vi "Autonomous Independent.vi"   [LabVIEW 2011]
doc: "This VI is called when autonomous begins, and will automatically be terminated when autonomous ends. You can carry out timed or sensor driven robot movement independently without needing to return to the caller."
uses:
  Robot Global Data.vi
types:
  T1 = typedef "WPI_JoystickDevRef.ctl" = cluster{"Device":T2}
  T2 = typedef "WPI_JoystickDeviceEnum.ctl" = enum16{"USB 1", "USB 2", "USB 3", "USB 4", "Kinect 1", "Kinect 2"}
  T3 = cluster{"axis 1 (x)":dbl, "axis 2 (y)":dbl, "axis 3 (throttle)":dbl, "axis 4":dbl, "axis 5":dbl, "axis 6":dbl}
  T4 = typedef "WPI_RobotDriveDevRef.ctl" = cluster{"DevStatus":errorcluster, "Motors[]":T5[], "Square Inputs":bool, "Max Output":dbl, "Isochronous":bool}
  T5 = typedef "WPI_MotorControlDeviceRef.ctl" = cluster{"DeviceStatus":errorcluster, "Type":enum16{"PWM", "CAN"}, "PWM":cluster{"Digital Module":T6, "PWM Channel":T7, "DeadBand":T8}, "CAN":cluster{"Device Number":u8, "Control Mode":T9, "Semaphore":T10, "Max Vout":dbl}, "Invert":bool, "TransformRef":T11, "InvTransformRef":T11}
  T6 = typedef "FPGA_TypedefDigitalModule.ctl" = enum16{"Digital Module 1", "Digital Module 2"}
  T7 = typedef "FPGA_DIOPWMChannel.ctl" = enum8{"PWM 1", "PWM 2", "PWM 3", "PWM 4", "PWM 5", "PWM 6", "PWM 7", "PWM 8", "PWM 9", "PWM 10", "Invalid"}
  T8 = typedef "WPI_PWMDeadband.ctl" = cluster{"Name":string, "maxPositivePwm":i32, "minPositivePwm":i32, "centerPwm":i32, "maxNegativePwm":i32, "minNegativePwm":i32, "angularRange":u16}
  T9 = typedef "WPI_CANJaguar_ControlMode.ctl" = enum8{"Percent VBus", "Current", "Speed", "Position", "Voltage"}
  T10 = typedef "Semaphore RefNum" = refnum<k1>
  T11 = typedef "WPI_PWMTransform_ConPane.ctl" = refnum<vi>
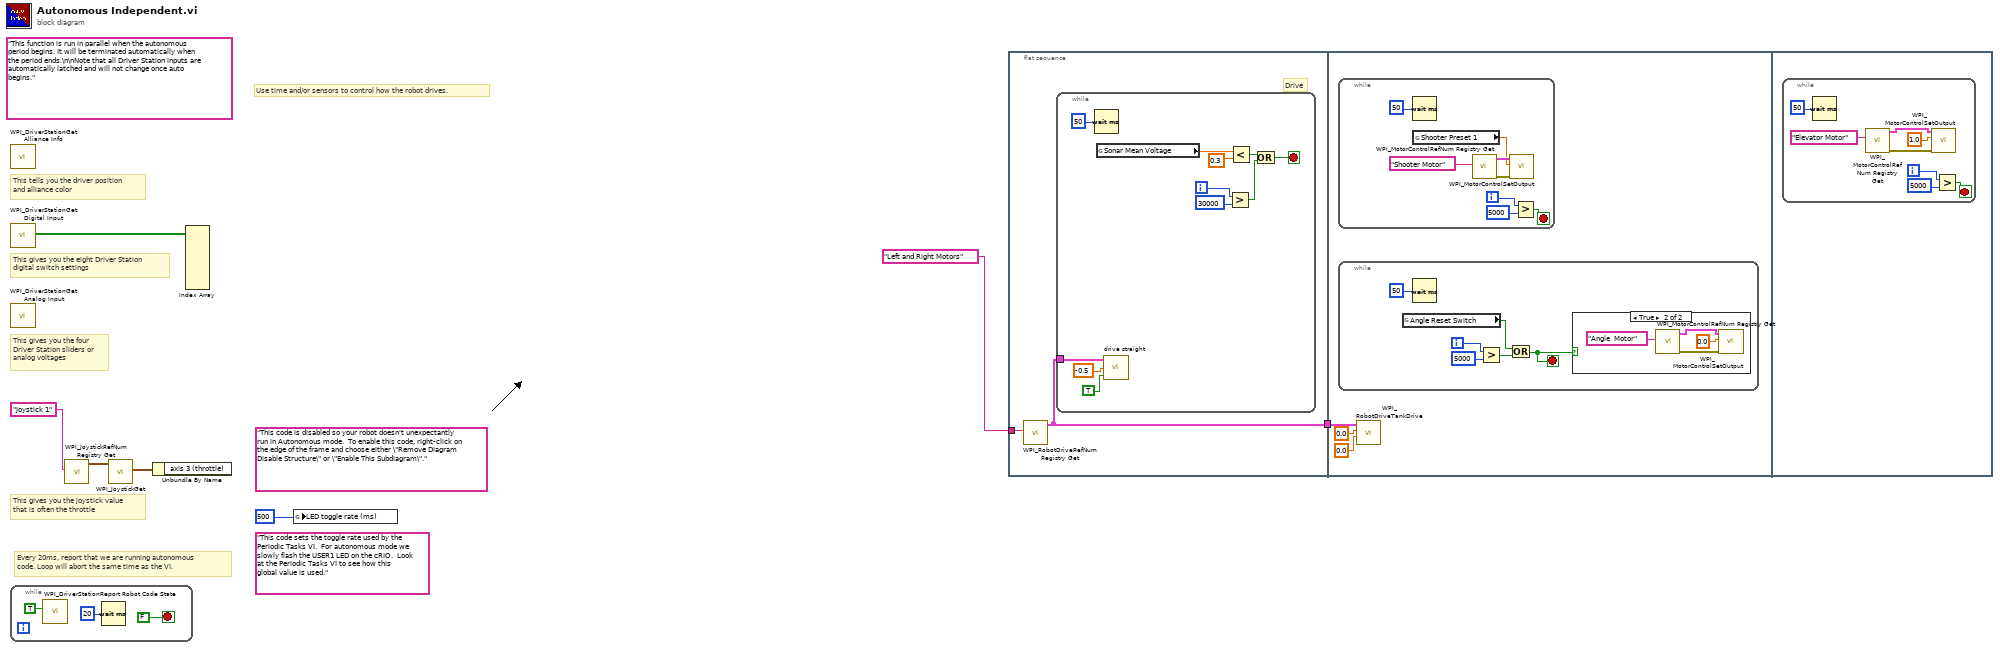
[diagram p0: block diagram]
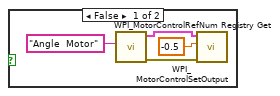
[diagram p2: hidden frame]
diagram:
  (unwired) "This code sets the toggle rate used by the Periodic Tasks VI.  For autonomous mode we slowly flash the USER1 LED on the cRIO.  Look at the Periodic Tasks VI to see how this global value is used."
  (unwired) "This code is disabled so your robot doesn't unexpectantly run in Autonomous mode.  To enable this code, right-click on the edge of the frame and choose either \"Remove Diagram Disable Structure\" or \"Enable This Subdiagram\"."
  (unwired) "This function is run in parallel when the autonomous period begins. It will be terminated automatically when the period ends.\n\nNote that all Driver Station inputs are automatically latched and will not change once auto begins."
  # "Every 20ms, report that we are running autonomous\ncode. Loop will abort the same time as the VI."
  # "This gives you the joystick value\nthat is often the throttle"
  # "Use time and/or sensors to control how the robot drives."
  # "This tells you the driver position\nand alliance color"
  # "This gives you the eight Driver Station\ndigital switch settings"
  # "This gives you the four\nDriver Station sliders or\nanalog voltages"
  n1 = while {
    stop <- FALSE stop-if-true
    n2 = call <vilib>:"WPI_DriverStationReport Robot Code State.vi"("Autonomous"=TRUE) -> ()  [unwired: 10 in, 1 out]
    n3 = Wait (ms)(milliseconds to wait=u32 20) -> ()  [unwired: 1 out]
  }
  n4 = call <vilib>:"WPI_DriverStationGet Alliance Info.vi"() -> ()  [unwired: 12 out]
  n5 = call <vilib>:"WPI_DriverStationGet Digital Input.vi"() -> ("Driver Station Digital Input (1-8)"=w7:bool[])  [unwired: 11 out]
  n6 = call <vilib>:"WPI_DriverStationGet Analog Input.vi"() -> ()  [unwired: 12 out]
  n7 = call <vilib>:"WPI_JoystickRefNum Registry Get.vi"("refnum name"="Joystick 1") -> ("JoystickDevRef"=w4:T1)  [unwired: 1 in, 9 out]
  n8 = call <vilib>:"WPI_JoystickGet.vi"("JoystickDevRef"=w4) -> ("Axes"=w5:T3)  [unwired: 1 in, 5 out]
  n9 = Unbundle By Name(w5) -> ()  [unwired: 1 out]
  n10 = Index Array(array=w7) -> ()  [unwired: 8 in, 8 out]
  n11 = global write "Robot Global Data.vi" "LED toggle rate (ms)"(u32 500 ("LED ms toggle rate")) -> ()
  n12 = flat-sequence {
    tunnel: "Left and Right Motors" ("refnum name") -> [w12]
    tunnel: [w11] -> w1
    tunnel: w1 -> [w25]
    frame #0 {
      # "Drive"
      n13 = call <vilib>:"WPI_RobotDriveRefNum Registry Get.vi"("refnum name"=w12) -> ("RobotDriveDevRef"=w11:T4)  [unwired: 1 in, 9 out]
      n14 = while {
        tunnel: w11 -> [w15]
        i -> [w20]
        stop <- w22 stop-if-true
        n15 = Wait (ms)(milliseconds to wait=50) -> ()  [unwired: 1 out]
        n16 = global read "Robot Global Data.vi" "Sonar Mean Voltage"() -> (w17:dbl)
        n17 = call "drive straight.vi"("Reverse"=TRUE, "Speed"=-0.5, "RobotDriveDevRef"=w15) -> ()  [unwired: 1 in]
        n18 = Greater?(x=w20, y=30000) -> (0:w23:bool)
        n19 = Less?(x=w17, y=0.3) -> (x < y?=w16:bool)
        n20 = Or(x=w16, y=w23) -> (x .or. y?=w22:bool)
      }
    }
    frame #1 {
      n21 = while {
        i -> [w43]
        stop <- w41 stop-if-true
        n22 = Wait (ms)(milliseconds to wait=50) -> ()  [unwired: 1 out]
        n23 = global read "Robot Global Data.vi" "Shooter Preset 1"() -> (w45:dbl)
        n24 = call <vilib>:"WPI_MotorControlRefNum Registry Get.vi"("refnum name"="Shooter Motor") -> ("error out"=w47:errorcluster, "MotorControlDevRef"=w46:T5)  [unwired: 9 in]
        n25 = call <vilib>:"WPI_MotorControlSetOutput.vi"("error in (no error)"=w47, "Output"=w45, "MotorControlDevRef"=w46) -> ()  [unwired: 7 in, 2 out]
        n26 = Greater?(x=w43, y=5000) -> (0:w41:bool)
      }
      n27 = while {
        i -> [w30]
        stop <- w27 stop-if-true
        n28 = global read "Robot Global Data.vi" "Angle Reset Switch"() -> (w28:bool)
        n29 = Wait (ms)(milliseconds to wait=50) -> ()  [unwired: 1 out]
        n30 = Greater?(x=w30, y=5000) -> (0:w29:bool)
        n31 = Or(x=w28, y=w29) -> (x .or. y?=w27:bool)
        n32 = case shown="True" w27 {
          frame False {
            n33 = call <vilib>:"WPI_MotorControlRefNum Registry Get.vi"("refnum name"="Angle  Motor") -> ("error out"=w35:errorcluster, "MotorControlDevRef"=w34:T5)  [unwired: 9 in]
            n34 = call <vilib>:"WPI_MotorControlSetOutput.vi"("error in (no error)"=w35, "Output"=-0.5, "MotorControlDevRef"=w34) -> ()  [unwired: 7 in, 2 out]
          }
          frame True {
            n35 = call <vilib>:"WPI_MotorControlRefNum Registry Get.vi"("refnum name"="Angle  Motor") -> ("error out"=w38:errorcluster, "MotorControlDevRef"=w39:T5)  [unwired: 9 in]
            n36 = call <vilib>:"WPI_MotorControlSetOutput.vi"("error in (no error)"=w38, "Output"=0.0, "MotorControlDevRef"=w39) -> ()  [unwired: 7 in, 2 out]
          }
        }
      }
      n37 = call <vilib>:"WPI_RobotDriveTankDrive.vi"("Right axis value"=0.0 ("X axis value"), "Left axis value"=0.0 ("X axis value"), "RobotDriveDevRef"=w25) -> ()  [unwired: 7 in, 2 out]
    }
    frame #2 {
      n38 = while {
        i -> [w51]
        stop <- w49 stop-if-true
        n39 = Wait (ms)(milliseconds to wait=50) -> ()  [unwired: 1 out]
        n40 = call <vilib>:"WPI_MotorControlRefNum Registry Get.vi"("refnum name"="Elevator Motor") -> ("error out"=w55:errorcluster, "MotorControlDevRef"=w54:T5)  [unwired: 9 in]
        n41 = call <vilib>:"WPI_MotorControlSetOutput.vi"("error in (no error)"=w55, "Output"=1.0, "MotorControlDevRef"=w54) -> ()  [unwired: 7 in, 2 out]
        n42 = Greater?(x=w51, y=5000) -> (0:w49:bool)
      }
    }
  }
